vi "ProgramableSharedVar.vi"(7 "Data Type":T1, 8 "error in (no error)":errorcluster, 9 "String":string, 10 "ro/r/w":T2=enum."Read Only", 11 "Data in":i64) -> (0 "error out":errorcluster, 1 "TimeStamp":timestamp, 2 "Data out":i64, 3 "PDO Path":refnum<k21>)   [LabVIEW 2016, in "Motor Base.lvlib" / "Motor Base.lvclass"]
uses:
  Motor Base.lvclass
  AccessType.ctl
  Data Type.ctl
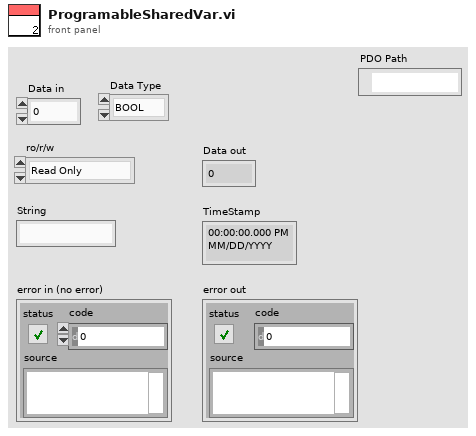
[diagram p1: front panel]
types:
  T1 = typedef "Motor Base.lvlib/Motor Base.lvclass/Data Type.ctl" = enum16{"BOOL", "I16", "I32", "I8", "OS", "U16", "U32", "U8", "VS"}
  T2 = typedef "Motor Base.lvlib/Motor Base.lvclass/AccessType.ctl" = enum16{"Write", "Read", "Read Only"}
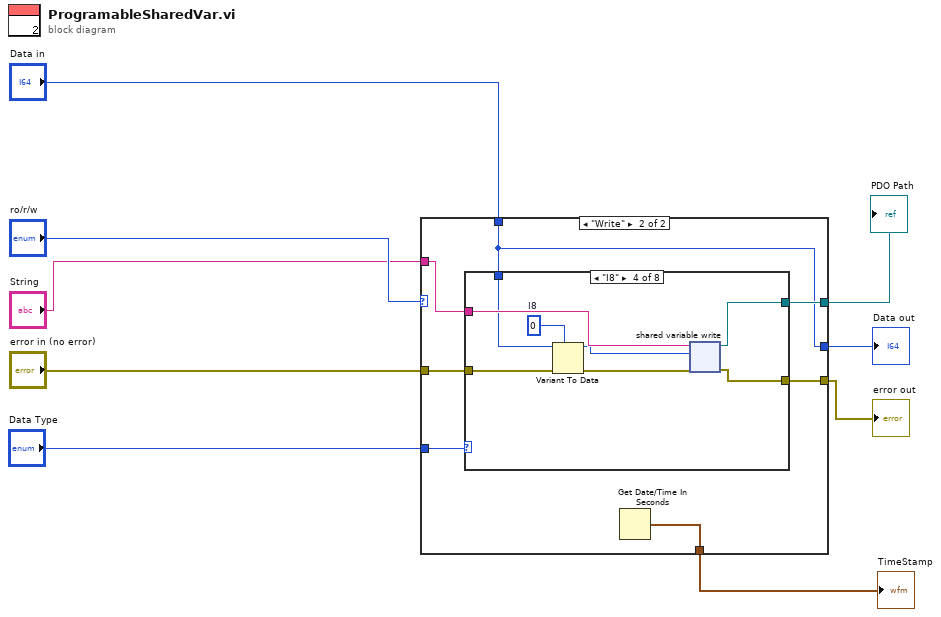
[diagram p0: block diagram]
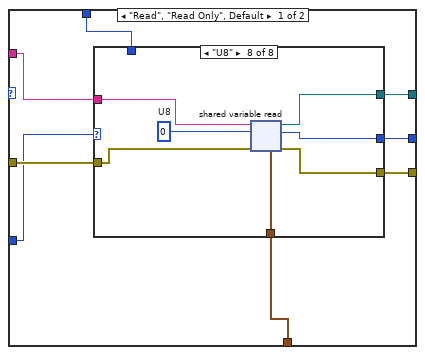
[diagram p2: hidden frame]
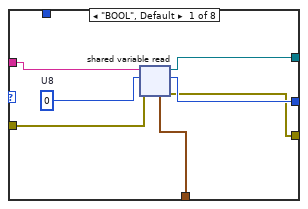
[diagram p3: hidden frame]
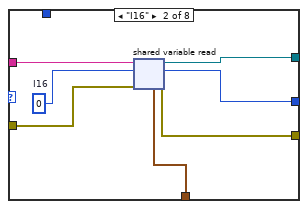
[diagram p4: hidden frame]
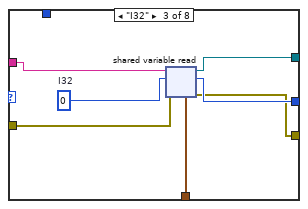
[diagram p5: hidden frame]
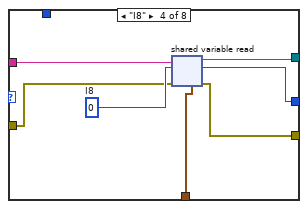
[diagram p6: hidden frame]
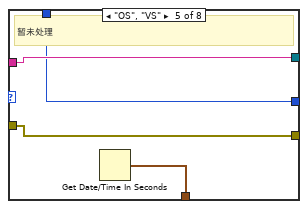
[diagram p7: hidden frame]
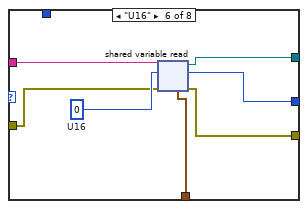
[diagram p8: hidden frame]
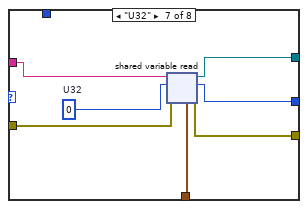
[diagram p9: hidden frame]
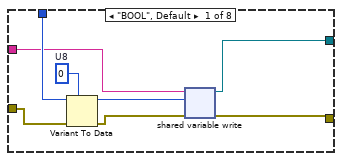
[diagram p10: hidden frame]
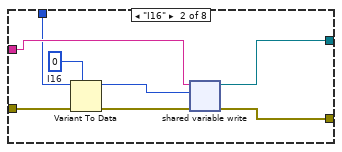
[diagram p11: hidden frame]
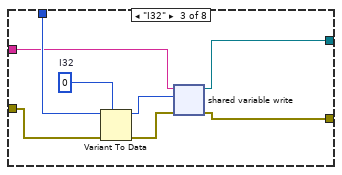
[diagram p12: hidden frame]
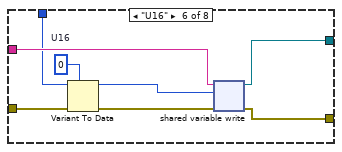
[diagram p14: hidden frame]
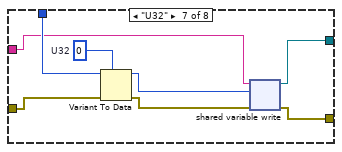
[diagram p15: hidden frame]
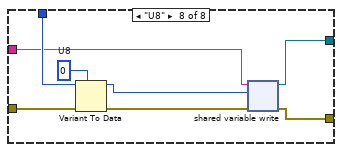
[diagram p16: hidden frame]
diagram:
  n1 = case shown="\"Write\"" "ro/r/w" {
    tunnel: "String" -> [w17 w77]
    tunnel: [w16 w76] -> w1
    tunnel: [w15 w72] -> w6
    tunnel: "error in (no error)" -> [w14 w75]
    tunnel: [w13 w74] -> w8
    tunnel: [w11 w73] -> w7
    tunnel: "Data in" -> [w10 w72]
    tunnel: "Data Type" -> [w12 w71]
    frame "Read", "Read Only", Default {
      n2 = case shown="\"U8\"" w12 {
        tunnel: w17 -> [w24 w31 w38 w44 w49 w55 w62 w69]
        tunnel: [w22 w30 w37 w43 w49 w54 w61 w68] -> w16
        tunnel: [w21 w29 w35 w39 w47 w51 w60 w67] -> w15
        tunnel: w14 -> [w20 w28 w34 w42 w46 w53 w59 w66]
        tunnel: [w19 w27 w32 w40 w46 w52 w58 w65] -> w13
        tunnel: [w18 w25 w33 w41 w48 w50 w57 w64] -> w11
        tunnel: w10 -> [_ _ _ _ w47 _ _ _]
        frame "BOOL", Default {
          w23 = u8 0  # U8
          n3 = shared-variable-read ("Scanned Variable Read")(w24, w20, w23) -> (w22:refnum<k21>, w19:errorcluster, w21:u8, w18:timestamp)
        }
        frame "I16" {
          w26 = i16 0  # I16
          n4 = shared-variable-read ("Scanned Variable Read")(w31, w28, w26) -> (w30:refnum<k21>, w27:errorcluster, w29:i16, w25:timestamp)
        }
        frame "I32" {
          w36 = 0  # I32
          n5 = shared-variable-read ("Scanned Variable Read")(w38, w34, w36) -> (w37:refnum<k21>, w32:errorcluster, w35:i32, w33:timestamp)
        }
        frame "I8" {
          w45 = i8 0  # I8
          n6 = shared-variable-read ("Scanned Variable Read")(w44, w42, w45) -> (w43:refnum<k21>, w40:errorcluster, w39:i8, w41:timestamp)
        }
        frame "OS", "VS" {
          # "暂未处理"
          n7 = Get Date/Time In Seconds() -> (seconds since 1Jan1904=w48:timestamp)
        }
        frame "U16" {
          w56 = u16 0  # U16
          n8 = shared-variable-read ("Scanned Variable Read")(w55, w53, w56) -> (w54:refnum<k21>, w52:errorcluster, w51:u16, w50:timestamp)
        }
        frame "U32" {
          w63 = u32 0  # U32
          n9 = shared-variable-read ("Scanned Variable Read")(w62, w59, w63) -> (w61:refnum<k21>, w58:errorcluster, w60:u32, w57:timestamp)
        }
        frame "U8" {
          w70 = u8 0  # U8
          n10 = shared-variable-read ("Scanned Variable Read")(w69, w66, w70) -> (w68:refnum<k21>, w65:errorcluster, w67:u8, w64:timestamp)
        }
      }
    }
    frame "Write" {
      n11 = case shown="\"I8\"" w71 {
        tunnel: w77 -> [w82 w93 w97 w105 w110 w116 w122 w129]
        tunnel: [w81 w92 w94 w106 w110 w112 w121 w128] -> w76
        tunnel: w75 -> [w80 w90 w99 w109 w111 w118 w125 w135]
        tunnel: [w78 w91 w95 w107 w111 w117 w120 w133] -> w74
        tunnel: w72 -> [w84 w88 w100 w103 _ w114 w127 w131]
        frame "BOOL", Default {
          w85 = u8 0  # U8
          n12 = Variant To Data(error in=w80, type=w85, Variant=w84) -> (data=w83:u8, error out=w79:errorcluster)
          n13 = shared-variable-write ("Scanned Variable Write")(w82, w79, w83) -> (w81:refnum<k21>, w78:errorcluster)
        }
        frame "I16" {
          w87 = i16 0  # I16
          n14 = Variant To Data(error in=w90, type=w87, Variant=w88) -> (data=w86:i16, error out=w89:errorcluster)
          n15 = shared-variable-write ("Scanned Variable Write")(w93, w89, w86) -> (w92:refnum<k21>, w91:errorcluster)
        }
        frame "I32" {
          w101 = 0  # I32
          n16 = Variant To Data(error in=w99, type=w101, Variant=w100) -> (data=w98:i32, error out=w96:errorcluster)
          n17 = shared-variable-write ("Scanned Variable Write")(w97, w96, w98) -> (w94:refnum<k21>, w95:errorcluster)
        }
        frame "I8" {
          w104 = i8 0  # I8
          n18 = Variant To Data(error in=w109, type=w104, Variant=w103) -> (data=w102:i8, error out=w108:errorcluster)
          n19 = shared-variable-write ("Scanned Variable Write")(w105, w108, w102) -> (w106:refnum<k21>, w107:errorcluster)
        }
        frame "OS", "VS" {
        }
        frame "U16" {
          w115 = u16 0  # U16
          n20 = Variant To Data(error in=w118, type=w115, Variant=w114) -> (data=w113:u16, error out=w119:errorcluster)
          n21 = shared-variable-write ("Scanned Variable Write")(w116, w119, w113) -> (w112:refnum<k21>, w117:errorcluster)
        }
        frame "U32" {
          w126 = u32 0  # U32
          n22 = Variant To Data(error in=w125, type=w126, Variant=w127) -> (data=w123:u32, error out=w124:errorcluster)
          n23 = shared-variable-write ("Scanned Variable Write")(w122, w124, w123) -> (w121:refnum<k21>, w120:errorcluster)
        }
        frame "U8" {
          w132 = u8 0  # U8
          n24 = Variant To Data(error in=w135, type=w132, Variant=w131) -> (data=w130:u8, error out=w134:errorcluster)
          n25 = shared-variable-write ("Scanned Variable Write")(w129, w134, w130) -> (w128:refnum<k21>, w133:errorcluster)
        }
      }
      n26 = Get Date/Time In Seconds() -> (seconds since 1Jan1904=w73:timestamp)
    }
  }
  "error out" <- w8
  "TimeStamp" <- w7
  "Data out" <- w6
  "PDO Path" <- w1
